vi "Find Background Pixel Average (SubVI).vi"(11 "Refnum in":T1) -> (3 "BG Average":sgl)   [LabVIEW 2014]
uses:
  <vilib>/vision/Image Controls.llb/IMAQ Image.ctl
  <vilib>/vision/NI_Vision_Development_Module.lvlib
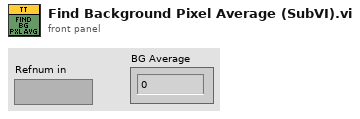
[diagram p1: front panel]
types:
  T1 = typedef "IMAQ Image.ctl" = refnum<image>
  T2 = cluster{"Mean Value":sgl, "Standard Variation":sgl, "Minimal Value":sgl, "Maximal Value":sgl, "Area (calibrated)":sgl, "Area (pixels)":u32, "%":sgl, "Calibration Valid":bool}
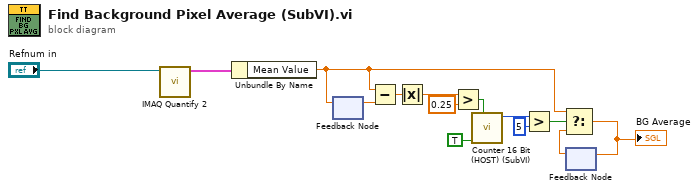
[diagram p0: block diagram]
diagram:
  n1 = call "IMAQ Quantify 2"("Image"="Refnum in") -> ("Global Report"=w2:T2)  [unwired: 8 in, 2 out]
  n2 = Unbundle By Name(w2) -> ("Mean Value"=w11:sgl)
  n3 = feedback #1() -> (w3:sgl)  [unwired: 1 in]
  n4 = feedback-in #1(w11) -> ()
  n5 = Subtract(x=w11, y=w3) -> (x-y=w4:sgl)
  n6 = Absolute Value(x=w4) -> (abs(x)=w14:sgl)
  n7 = Greater?(x=w14, y=sgl 0.25) -> (0:w5:bool)
  n8 = call "Counter 16 Bit (HOST) (SubVI).vi"("RESET"=w5, "Enable"=TRUE) -> ("Count"=w6:u16)  [unwired: 7 in, 2 out]
  n9 = Greater?(x=w6, y=u16 5) -> (0:w10:bool)
  n10 = feedback #2() -> (w12:sgl)  [unwired: 1 in]
  n11 = Select(t=w11, s=w10, f=w12) -> (s? t:f=w13:sgl)
  "BG Average" <- w13
  n12 = feedback-in #2(w13) -> ()
